vi "Drive Controller.vi"(8 "error in":errorcluster) -> ()   [LabVIEW 2020]
doc: "This VI executes continuously carrying out the current operation and responding to updates or new operation requests. It will often contain the timing or control code that is difficult to place directly in TeleOp. This VI generally opens all sensors and motors and isolates the rest of the robot code from knowing implementation details of how the operations are carried out."
uses:
  <vilib>/Rock Robotics/WPI/Framework/Completion Status.ctl
  Drive Setpoints.ctl
  Drive Operations.ctl
  <vilib>/Rock Robotics/WPI/SafetyOutput/WPI_SafetyOutputConfigMenu.ctl
  <vilib>/Rock Robotics/WPI/RobotDrive/WPI_RobotDriveOpen2MotorWithExistingMotors.vi
  <vilib>/Rock Robotics/Network Tables/NT Write Numeric Array.vi
  <vilib>/Rock Robotics/WPI/ThirdParty/REV Robotics/REVLib/Typedef/Spark MAX Motor Type.ctl
  <vilib>/Rock Robotics/WPI/ThirdParty/REV Robotics/REVLib/Typedef/Spark MAX Idle Mode.ctl
panel:
  in  "Interactive Values":T1
  in  "Buttons":cluster{"Execute Cmd":bool, "Abort Cmd":bool}
  out "Command Timing":cluster{"Start Time (ms)":u32, "Iterations":i32}
  out "Status":T3
  out "Setpoints":T4(graph)
  out "Current\nCmd":string
  # "Tip: The graph shows the motor setpoints. It may also be helpful to observe inputs and sensor values.\nYou may also want to display tuning or debugging controls."
  # "Interactive Command: You may fill in the settings for a command\nand schedule it with the Execute button. You can observe and abort\nany command while fine tuning the code for the controller."
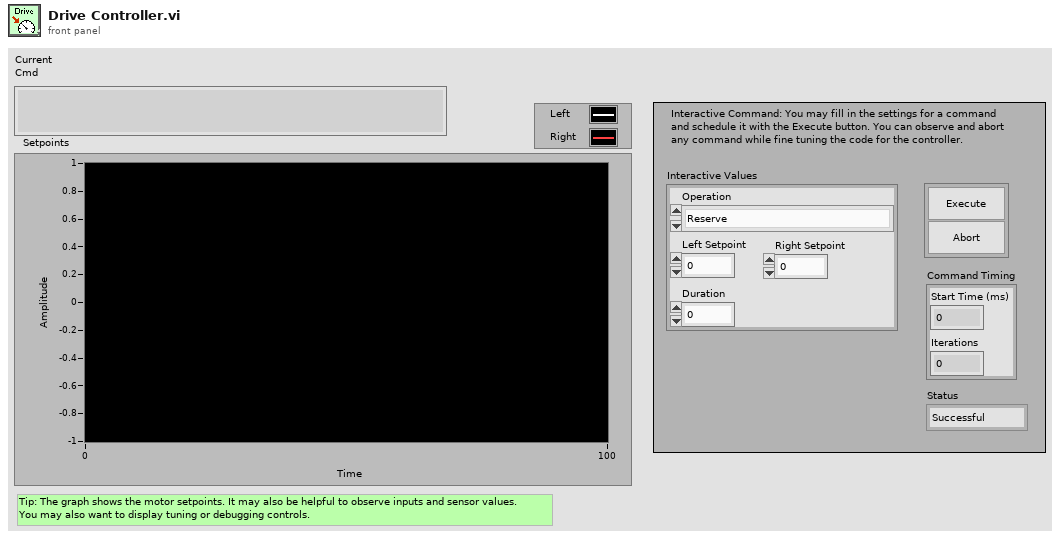
[diagram p1: front panel]
types:
  T1 = typedef "Drive Setpoints.ctl" = cluster{"Operation":T2, "Left Setpoint":dbl, "Right Setpoint":dbl, "Duration":dbl}
  T2 = typedef "Drive Operations.ctl" = enum16{"Reserve", "Read Current", "Immediate", "Drive for Time", "Drive for Distance"}
  T3 = typedef "Completion Status.ctl" = enum16{"Successful", "Aborted", "Incomplete"}
  T4 = cluster{"Left Setpoint":dbl, "Right Setpoint":dbl}
  T5 = typedef "WPI_SafetyOutputConfigMenu.ctl" = enum16{"Enable", "Disable"}
  T6 = typedef "Spark MAX Motor Type.ctl" = enum16{"Brushed", "Brushless"}
  T7 = typedef "Spark MAX Idle Mode.ctl" = enum16{"Coast", "Brake"}
  T8 = typedef "WPI_MotorControlDeviceRef.ctl" = cluster{"DeviceStatus":errorcluster, "Type":T9, "PWM":cluster{"PWM Channel":T10, "DeadBand":T11}, "CAN":cluster{"Device Number":u8, "SetOutput VI Ref":variant, "GetOutput VI Ref":variant, "Enable VI Ref":variant, "Disable VI Ref":variant, "Data":variant}, "Invert":bool, "DIO PWM":cluster{"PWM \"Enable\" Channel":T10, "DIOChannel":T12, "PWM Rate":dbl}}
  T9 = typedef "WPI_MotorControlType.ctl" = enum16{"PWM", "CAN", "DIO PWM"}
  T10 = typedef "FPGA_DIOPWMChannel.ctl" = enum8{"PWM 0", "PWM 1", "PWM 2", "PWM 3", "PWM 4", "PWM 5", "PWM 6", "PWM 7", "PWM 8", "PWM 9", "PWM MXP 0", "PWM MXP 1", "PWM MXP 2", "PWM MXP 3", "PWM MXP 4", "PWM MXP 5", "PWM MXP 6", "PWM MXP 7", "PWM MXP 8", "PWM MXP 9", "Invalid"}
  T11 = typedef "WPI_PWMDeadband.ctl" = cluster{"Name":string, "maxPositivePwm":i32, "minPositivePwm":i32, "centerPwm":i32, "maxNegativePwm":i32, "minNegativePwm":i32, "angularRange":u16}
  T12 = typedef "FPGA_DIOChannel.ctl" = enum8{"DIO 0", "DIO 1", "DIO 2", "DIO 3", "DIO 4", "DIO 5", "DIO 6", "DIO 7", "DIO 8", "DIO 9", "DIO MXP 0", "DIO MXP 1", "DIO MXP 2", "DIO MXP 3", "DIO MXP 4", "DIO MXP 5", "DIO MXP 6", "DIO MXP 7", "DIO MXP 8", "DIO MXP 9", "DIO MXP 10", "DIO MXP 11", "DIO MXP 12", "DIO MXP 13", "DIO MXP 14", "DIO MXP 15", "SPI Port CS1", "SPI Port CS2", "SPI Port CS3", "SPI Port MISO", "SPI Port MOSI", "Invalid"}
  T13 = typedef "WPI_RobotDriveDevRef.ctl" = cluster{"DevStatus":errorcluster, "Motors[]":T8[], "Square Inputs":bool, "Max Output":dbl}
  T14 = typedef "Command Status Info.ctl" = cluster{"Name":string, "Status":T3, "notifier out":T15}
  T15 = typedef "Completion Notifier.ctl" = refnum<notifier>
  T16 = cluster{"SubSystem Data":T1, cluster{"Start Time (ms)":u32, "Iterations":i32}, cluster{"Command Info":T14, "Description":string, "Default Command":T1, "queue out":refnum<queue>, "Subsystem Name":string}}
  T17 = cluster{"SubSystem Data":T1, cluster{"Start Time (ms)":u32, "Iterations":i32}, "Default Command Arguments":cluster{"Command Info":T14, "Description":string, "Default Command":T1, "queue out":refnum<queue>, "Subsystem Name":string}}
  T18 = cluster{"Don't move motors while reserved":dbl, "Don't move motors while reserved":dbl}
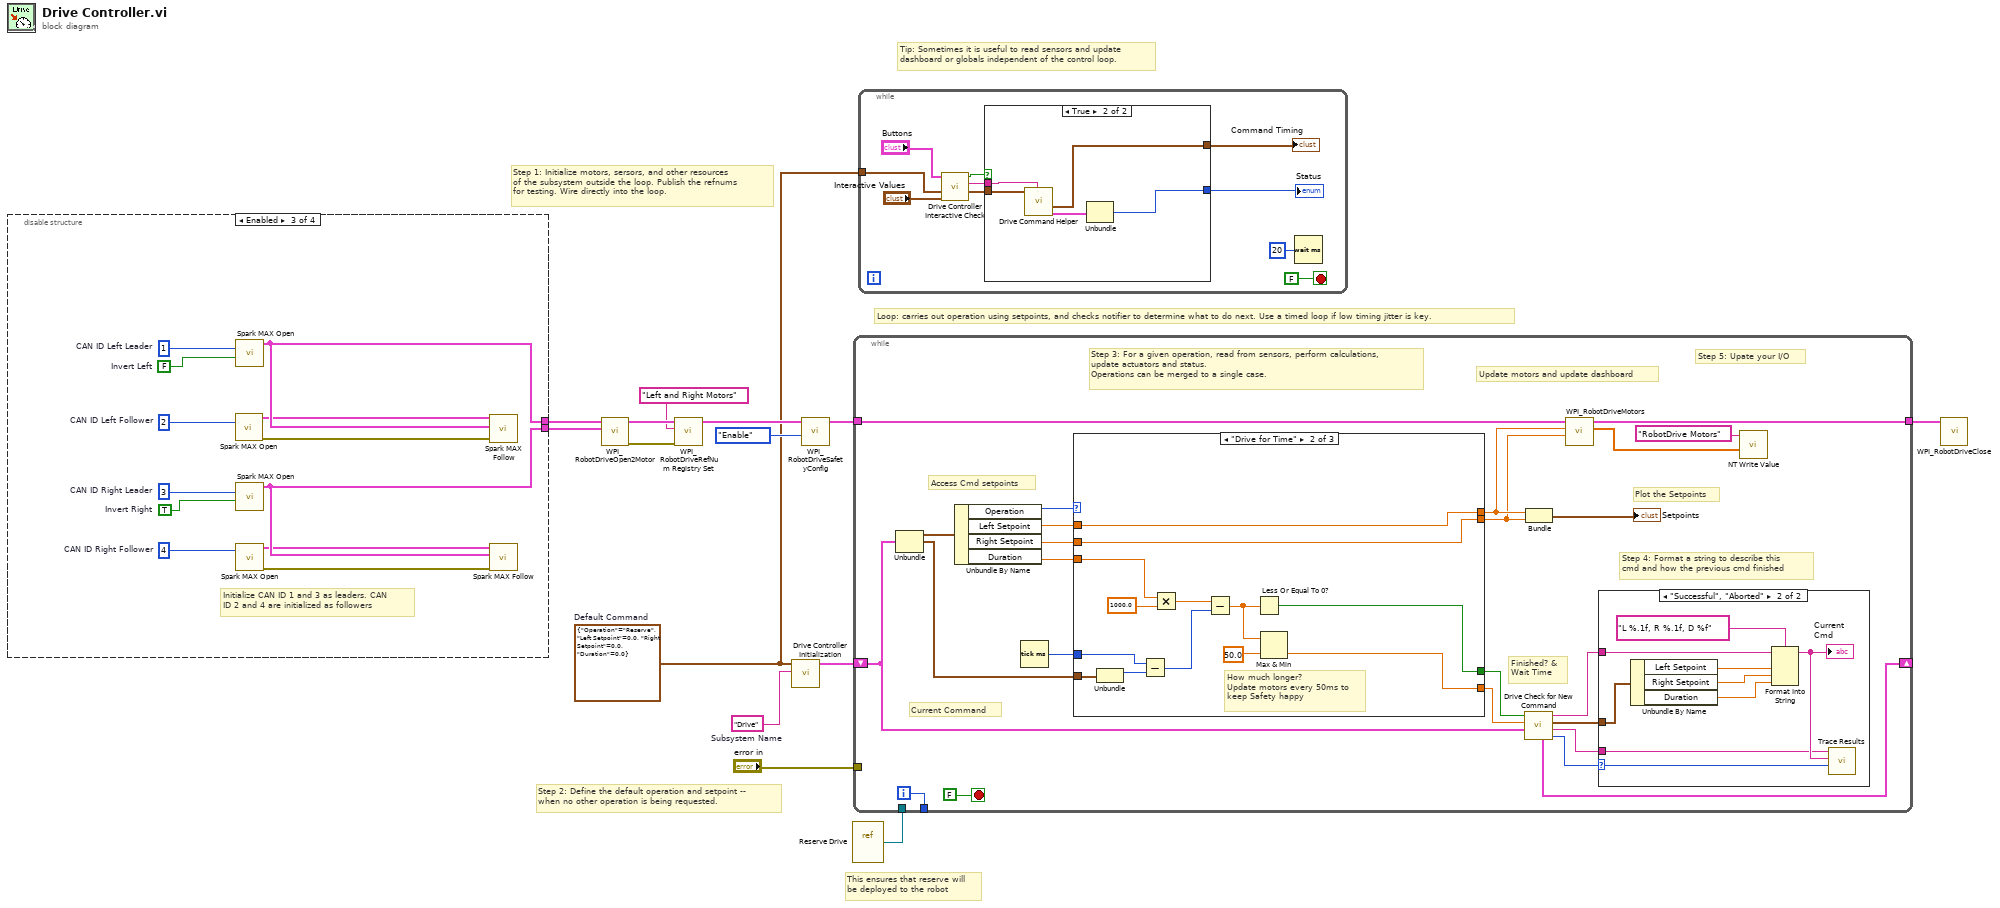
[diagram p0: block diagram]
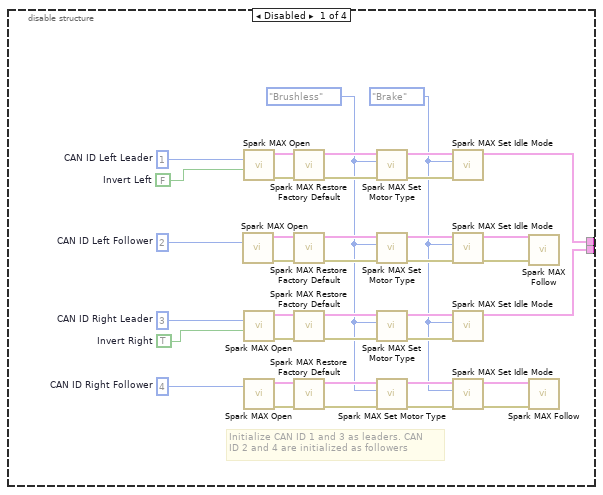
[diagram p2: hidden frame]
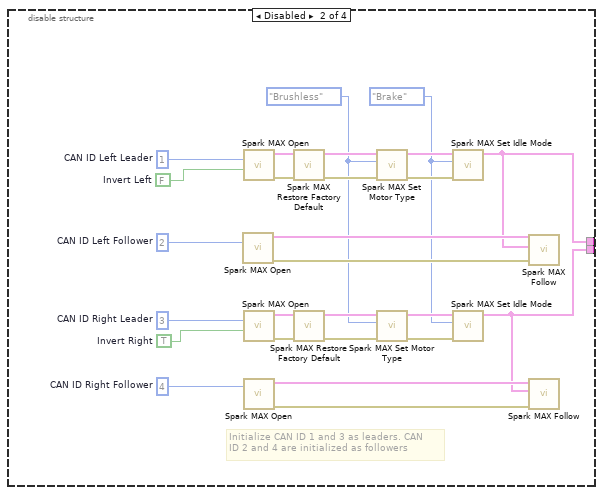
[diagram p3: hidden frame]
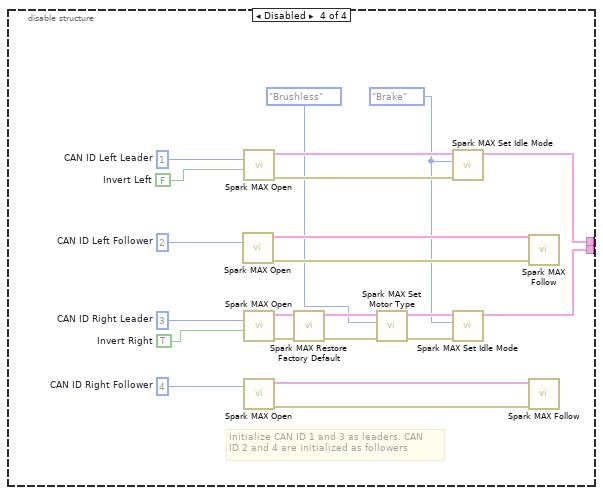
[diagram p4: hidden frame]
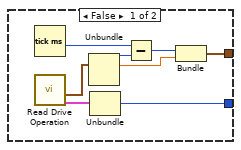
[diagram p5: hidden frame]
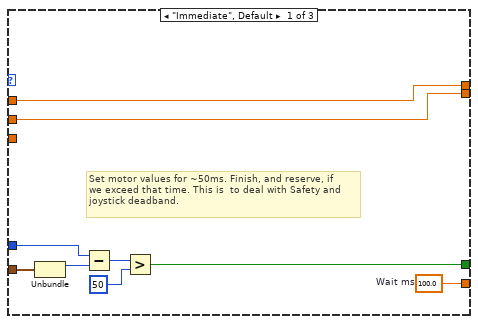
[diagram p7: hidden frame]
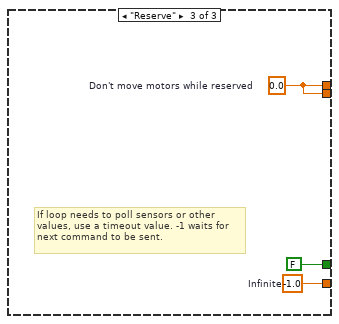
[diagram p8: hidden frame]
diagram:
  w4 = T1 {"Operation"=enum."Reserve", "Left Setpoint"=0.0, "Right Setpoint"=0.0, "Duration"=0.0}  # Default Command
  w14 = "Drive"  # Subsystem Name
  # "This ensures that reserve will\nbe deployed to the robot"
  # "Tip: Sometimes it is useful to read sensors and update\ndashboard or globals independent of the control loop."
  # "Step 2: Define the default operation and setpoint --\nwhen no other operation is being requested."
  # "Step 1: Initialize motors, sersors, and other resources\nof the subsystem outside the loop. Publish the refnums\nfor testing. Wire directly into the loop."
  # "Loop: carries out operation using setpoints, and checks notifier to determine what to do next. Use a timed loop if low timing jitter is key."
  n1 = disable-structure shown="Enabled" {
    disable-tunnel: [w22 w56 w86 w94] -> w3
    disable-tunnel: [w21 w55 w83 w93] -> w2
    frame Disabled {
      w23 = Spark_MAX_Idle_Mode."Brake" ("Idle Mode")
      w32 = Spark_MAX_Motor_Type."Brushless" ("Motor Type")
      w20 = FALSE  # Invert Left
      w19 = TRUE  # Invert Right
      w50 = u8 3  # CAN ID Right Leader
      w49 = u8 4  # CAN ID Right Follower
      w51 = u8 1  # CAN ID Left Leader
      w52 = u8 2  # CAN ID Left Follower
      # "Initialize CAN ID 1 and 3 as leaders. CAN \nID 2 and 4 are initialized as followers"
      n2 = call <vilib>:"Spark MAX Open.vi"("Device Number"=w52) -> ("error out"=w46:errorcluster, "MotorControlDeviceRef"=w45:T8)  [unwired: 9 in]
      n3 = call <vilib>:"Spark MAX Open.vi"("Invert"=w20, "Device Number"=w51) -> ("error out"=w48:errorcluster, "MotorControlDeviceRef"=w47:T8)  [unwired: 8 in]
      n4 = call <vilib>:"Spark MAX Open.vi"("Invert"=w19, "Device Number"=w50) -> ("error out"=w44:errorcluster, "MotorControlDeviceRef"=w43:T8)  [unwired: 8 in]
      n5 = call <vilib>:"Spark MAX Open.vi"("Device Number"=w49) -> ("error out"=w42:errorcluster, "MotorControlDeviceRef"=w41:T8)  [unwired: 9 in]
      n6 = call <vilib>:"Spark MAX Restore Factory Default.vi"("error in"=w48, "MotorControlDeviceRef"=w47) -> ("error out"=w40:errorcluster, "MotorControlDeviceRef"=w39:T8)  [unwired: 8 in]
      n7 = call <vilib>:"Spark MAX Restore Factory Default.vi"("error in"=w46, "MotorControlDeviceRef"=w45) -> ("error out"=w38:errorcluster, "MotorControlDeviceRef"=w37:T8)  [unwired: 8 in]
      n8 = call <vilib>:"Spark MAX Restore Factory Default.vi"("error in"=w44, "MotorControlDeviceRef"=w43) -> ("error out"=w36:errorcluster, "MotorControlDeviceRef"=w35:T8)  [unwired: 8 in]
      n9 = call <vilib>:"Spark MAX Restore Factory Default.vi"("error in"=w42, "MotorControlDeviceRef"=w41) -> ("error out"=w34:errorcluster, "MotorControlDeviceRef"=w33:T8)  [unwired: 8 in]
      n10 = call <vilib>:"Spark MAX Set Motor Type.vi"("error in (no error)"=w40, "Motor Type"=w32, "MotorControlDevRef"=w39) -> ("error out"=w31:errorcluster, "MotorControlDeviceRef"=w30:T8)  [unwired: 7 in]
      n11 = call <vilib>:"Spark MAX Set Motor Type.vi"("error in (no error)"=w38, "Motor Type"=w32, "MotorControlDevRef"=w37) -> ("error out"=w29:errorcluster, "MotorControlDeviceRef"=w28:T8)  [unwired: 7 in]
      n12 = call <vilib>:"Spark MAX Set Motor Type.vi"("error in (no error)"=w36, "Motor Type"=w32, "MotorControlDevRef"=w35) -> ("error out"=w27:errorcluster, "MotorControlDeviceRef"=w26:T8)  [unwired: 7 in]
      n13 = call <vilib>:"Spark MAX Set Motor Type.vi"("error in (no error)"=w34, "Motor Type"=w32, "MotorControlDevRef"=w33) -> ("error out"=w25:errorcluster, "MotorControlDeviceRef"=w24:T8)  [unwired: 7 in]
      n14 = call <vilib>:"Spark MAX Set Idle Mode.vi"("error in (no error)"=w31, "Idle Mode"=w23, "MotorControlDeviceRef in"=w30) -> ("MotorControlDeviceRef out"=w22:T8)  [unwired: 7 in, 1 out]
      n15 = call <vilib>:"Spark MAX Set Idle Mode.vi"("error in (no error)"=w29, "Idle Mode"=w23, "MotorControlDeviceRef in"=w28) -> ("error out"=w18:errorcluster, "MotorControlDeviceRef out"=w17:T8)  [unwired: 7 in]
      n16 = call <vilib>:"Spark MAX Set Idle Mode.vi"("error in (no error)"=w27, "Idle Mode"=w23, "MotorControlDeviceRef in"=w26) -> ("MotorControlDeviceRef out"=w21:T8)  [unwired: 7 in, 1 out]
      n17 = call <vilib>:"Spark MAX Set Idle Mode.vi"("error in (no error)"=w25, "Idle Mode"=w23, "MotorControlDeviceRef in"=w24) -> ("error out"=w16:errorcluster, "MotorControlDeviceRef out"=w15:T8)  [unwired: 7 in]
      n18 = call <vilib>:"Spark MAX Follow.vi"("error in (no error)"=w18, "MotorControlDeviceRef"=w17) -> ()  [unwired: 8 in, 2 out]
      n19 = call <vilib>:"Spark MAX Follow.vi"("error in (no error)"=w16, "MotorControlDeviceRef"=w15) -> ()  [unwired: 8 in, 2 out]
    }
    frame Disabled {
      w57 = Spark_MAX_Idle_Mode."Brake" ("Idle Mode")
      w62 = Spark_MAX_Motor_Type."Brushless" ("Motor Type")
      w54 = FALSE  # Invert Left
      w53 = TRUE  # Invert Right
      w76 = u8 3  # CAN ID Right Leader
      w75 = u8 4  # CAN ID Right Follower
      w77 = u8 1  # CAN ID Left Leader
      w78 = u8 2  # CAN ID Left Follower
      # "Initialize CAN ID 1 and 3 as leaders. CAN \nID 2 and 4 are initialized as followers"
      n20 = call <vilib>:"Spark MAX Open.vi"("Device Number"=w78) -> ("error out"=w68:errorcluster, "MotorControlDeviceRef"=w67:T8)  [unwired: 9 in]
      n21 = call <vilib>:"Spark MAX Open.vi"("Invert"=w54, "Device Number"=w77) -> ("error out"=w74:errorcluster, "MotorControlDeviceRef"=w73:T8)  [unwired: 8 in]
      n22 = call <vilib>:"Spark MAX Open.vi"("Invert"=w53, "Device Number"=w76) -> ("error out"=w72:errorcluster, "MotorControlDeviceRef"=w71:T8)  [unwired: 8 in]
      n23 = call <vilib>:"Spark MAX Open.vi"("Device Number"=w75) -> ("error out"=w64:errorcluster, "MotorControlDeviceRef"=w63:T8)  [unwired: 9 in]
      n24 = call <vilib>:"Spark MAX Restore Factory Default.vi"("error in"=w74, "MotorControlDeviceRef"=w73) -> ("error out"=w70:errorcluster, "MotorControlDeviceRef"=w69:T8)  [unwired: 8 in]
      n25 = call <vilib>:"Spark MAX Restore Factory Default.vi"("error in"=w72, "MotorControlDeviceRef"=w71) -> ("error out"=w66:errorcluster, "MotorControlDeviceRef"=w65:T8)  [unwired: 8 in]
      n26 = call <vilib>:"Spark MAX Set Motor Type.vi"("error in (no error)"=w70, "Motor Type"=w62, "MotorControlDevRef"=w69) -> ("error out"=w61:errorcluster, "MotorControlDeviceRef"=w60:T8)  [unwired: 7 in]
      n27 = call <vilib>:"Spark MAX Set Motor Type.vi"("error in (no error)"=w66, "Motor Type"=w62, "MotorControlDevRef"=w65) -> ("error out"=w59:errorcluster, "MotorControlDeviceRef"=w58:T8)  [unwired: 7 in]
      n28 = call <vilib>:"Spark MAX Set Idle Mode.vi"("error in (no error)"=w61, "Idle Mode"=w57, "MotorControlDeviceRef in"=w60) -> ("MotorControlDeviceRef out"=w56:T8)  [unwired: 7 in, 1 out]
      n29 = call <vilib>:"Spark MAX Set Idle Mode.vi"("error in (no error)"=w59, "Idle Mode"=w57, "MotorControlDeviceRef in"=w58) -> ("MotorControlDeviceRef out"=w55:T8)  [unwired: 7 in, 1 out]
      n30 = call <vilib>:"Spark MAX Follow.vi"("error in (no error)"=w68, "Master Controller"=w56, "MotorControlDeviceRef"=w67) -> ()  [unwired: 7 in, 2 out]
      n31 = call <vilib>:"Spark MAX Follow.vi"("error in (no error)"=w64, "Master Controller"=w55, "MotorControlDeviceRef"=w63) -> ()  [unwired: 7 in, 2 out]
    }
    frame Enabled {
      w80 = FALSE  # Invert Left
      w79 = TRUE  # Invert Right
      w88 = u8 3  # CAN ID Right Leader
      w87 = u8 4  # CAN ID Right Follower
      w89 = u8 1  # CAN ID Left Leader
      w90 = u8 2  # CAN ID Left Follower
      # "Initialize CAN ID 1 and 3 as leaders. CAN \nID 2 and 4 are initialized as followers"
      n32 = call <vilib>:"Spark MAX Open.vi"("Device Number"=w90) -> ("error out"=w85:errorcluster, "MotorControlDeviceRef"=w84:T8)  [unwired: 9 in]
      n33 = call <vilib>:"Spark MAX Open.vi"("Invert"=w80, "Device Number"=w89) -> ("MotorControlDeviceRef"=w86:T8)  [unwired: 8 in, 1 out]
      n34 = call <vilib>:"Spark MAX Open.vi"("Invert"=w79, "Device Number"=w88) -> ("MotorControlDeviceRef"=w83:T8)  [unwired: 8 in, 1 out]
      n35 = call <vilib>:"Spark MAX Open.vi"("Device Number"=w87) -> ("error out"=w82:errorcluster, "MotorControlDeviceRef"=w81:T8)  [unwired: 9 in]
      n36 = call <vilib>:"Spark MAX Follow.vi"("error in (no error)"=w85, "Master Controller"=w86, "MotorControlDeviceRef"=w84) -> ()  [unwired: 7 in, 2 out]
      n37 = call <vilib>:"Spark MAX Follow.vi"("error in (no error)"=w82, "Master Controller"=w83, "MotorControlDeviceRef"=w81) -> ()  [unwired: 7 in, 2 out]
    }
    frame Disabled {
      w95 = Spark_MAX_Idle_Mode."Brake" ("Idle Mode")
      w92 = FALSE  # Invert Left
      w91 = TRUE  # Invert Right
      w110 = u8 3  # CAN ID Right Leader
      w109 = u8 4  # CAN ID Right Follower
      w111 = u8 1  # CAN ID Left Leader
      w112 = u8 2  # CAN ID Left Follower
      # "Initialize CAN ID 1 and 3 as leaders. CAN \nID 2 and 4 are initialized as followers"
      n38 = call <vilib>:"Spark MAX Open.vi"("Device Number"=w112) -> ("error out"=w104:errorcluster, "MotorControlDeviceRef"=w103:T8)  [unwired: 9 in]
      n39 = call <vilib>:"Spark MAX Open.vi"("Invert"=w92, "Device Number"=w111) -> ("error out"=w106:errorcluster, "MotorControlDeviceRef"=w105:T8)  [unwired: 8 in]
      n40 = call <vilib>:"Spark MAX Open.vi"("Invert"=w91, "Device Number"=w110) -> ("error out"=w108:errorcluster, "MotorControlDeviceRef"=w107:T8)  [unwired: 8 in]
      n41 = call <vilib>:"Spark MAX Open.vi"("Device Number"=w109) -> ("error out"=w100:errorcluster, "MotorControlDeviceRef"=w99:T8)  [unwired: 9 in]
      n42 = call <vilib>:"Spark MAX Restore Factory Default.vi"("error in"=w108, "MotorControlDeviceRef"=w107) -> ("error out"=w102:errorcluster, "MotorControlDeviceRef"=w101:T8)  [unwired: 8 in]
      n43 = call <vilib>:"Spark MAX Set Motor Type.vi"("error in (no error)"=w102, "Motor Type"=Spark_MAX_Motor_Type."Brushless", "MotorControlDevRef"=w101) -> ("error out"=w97:errorcluster, "MotorControlDeviceRef"=w96:T8)  [unwired: 7 in]
      n44 = call <vilib>:"Spark MAX Set Idle Mode.vi"("error in (no error)"=w106, "Idle Mode"=w95, "MotorControlDeviceRef in"=w105) -> ("MotorControlDeviceRef out"=w94:T8)  [unwired: 7 in, 1 out]
      n45 = call <vilib>:"Spark MAX Set Idle Mode.vi"("error in (no error)"=w97, "Idle Mode"=w95, "MotorControlDeviceRef in"=w96) -> ("MotorControlDeviceRef out"=w93:T8)  [unwired: 7 in, 1 out]
      n46 = call <vilib>:"Spark MAX Follow.vi"("error in (no error)"=w104, "MotorControlDeviceRef"=w103) -> ()  [unwired: 8 in, 2 out]
      n47 = call <vilib>:"Spark MAX Follow.vi"("error in (no error)"=w100, "MotorControlDeviceRef"=w99) -> ()  [unwired: 8 in, 2 out]
    }
  }
  n48 = call-poly <vilib>:"WPI_RobotDriveOpen2Motor.vi"("Right Motor Dev Ref"=w2, "Left Motor Dev Ref"=w3) -> ("error out"=w11:errorcluster, "RobotDriveDevRef"=w13:T13)  [unwired: 3 in, 5 out]
  n49 = call <vilib>:"WPI_RobotDriveRefNum Registry Set.vi"("error in (no error)"=w11, "refnum name"="Left and Right Motors", "RobotDriveDevRef"=w13) -> ("RobotDriveDevRef"=w10:T13)  [unwired: 1 in, 7 out]
  n50 = call "Drive Controller Initialization.vi"("Subsystem Name"=w14, "Default Command"=w4) -> ("Current Command"=w6:T16)  [unwired: 9 in]
  n51 = call <vilib>:"WPI_RobotDriveSafetyConfig.vi"("mode"=WPI_SafetyOutputConfigMenu."Enable", "RobotDriveDevRef"=w10) -> ("RobotDriveDevRef"=w8:T13)  [unwired: 8 in, 1 out]
  n52 = vi-ref "Reserve Drive.vi"() -> (w5:refnum<vi>)
  n53 = while {
    shift-right: [w123] -> _
    shift-left: w6 -> [w116]
    tunnel: [w135] -> _
    tunnel: w8 -> [w131]
    tunnel: "error in" -> [_]
    tunnel: w5 -> [_]
    tunnel: [w115] -> w1
    i -> [w135]
    stop <- FALSE stop-if-true
    # "Step 5: Upate your I/O"
    # "Step 4: Format a string to describe this\ncmd and how the previous cmd finished"
    # "Current Command"
    # "Update motors and update dashboard"
    # "Plot the Setpoints"
    # "Access Cmd setpoints"
    # "Finished? &\nWait Time"
    # "Step 3: For a given operation, read from sensors, perform calculations,\nupdate actuators and status.\nOperations can be merged to a single case."
    n54 = Unbundle(w116) -> ("SubSystem Data"=w130:T1, w117:cluster{"Start Time (ms)":u32, "Iterations":i32})  [unwired: 1 out]
    n55 = Unbundle By Name(w130) -> ("Operation"=w129:T2, "Left Setpoint"=w128:dbl, "Right Setpoint"=w127:dbl, "Duration"=w126:dbl)
    n56 = Tick Count (ms)() -> (millisecond timer value=w125:u32)
    n57 = case shown="\"Drive for Time\"" w129 {
      tunnel: [w154 w155 w170] -> w122
      tunnel: [w147 w162 FALSE ("ignore previous (F)")] -> w121
      tunnel: w117 -> [w146 w164 _]
      tunnel: [w153 w161 w168] -> w133
      tunnel: [w152 w160 w168] -> w132
      tunnel: w128 -> [w153 w161 _]
      tunnel: w127 -> [w152 w160 _]
      tunnel: w126 -> [_ w159 _]
      tunnel: w125 -> [w148 w158 _]
      frame "Immediate", Default {
        w154 = 100.0  # Wait ms
        # "Set motor values for ~50ms. Finish, and reserve, if\nwe exceed that time. This is  to deal with Safety and\njoystick deadband."
        n58 = Unbundle(w146) -> ("Start Time (ms)"=w149:u32)  [unwired: 1 out]
        n59 = Subtract(x=w148, y=w149) -> (x-y=w150:u32)
        n60 = Greater?(x=w150, y=u8 50 ("Left Motor")) -> (0:w147:bool)
      }
      frame "Drive for Time" {
        # "How much longer?\nUpdate motors every 50ms to\nkeep Safety happy"
        n61 = Unbundle(w164) -> ("Start Time (ms)"=w163:u32)  [unwired: 1 out]
        n62 = Subtract(x=w158, y=w163) -> (x-y=w167:u32)
        n63 = Multiply(x=w159, y=1000.0) -> (x*y=w166:dbl)
        n64 = Subtract(x=w166, y=w167) -> (x-y=w157:dbl)
        n65 = Less Or Equal To 0?(x=w157) -> (x <= 0?=w162:bool)
        n66 = Max & Min(x=w157, y=50.0) -> (min(x,y)=w155:dbl)  [unwired: 1 out]
      }
      frame "Reserve" {
        w168 = 0.0  # Don't move motors while reserved
        w170 = -1.0  # Infinite
        # "If loop needs to poll sensors or other\nvalues, use a timeout value. -1 waits for\nnext command to be sent."
      }
    }
    n67 = call "Drive Check for New Command.vi"("input cluster"=w116, "Wait time (ms)"=w122, "Finished?"=w121) -> ("Completion"=w124:T3, "Subsystem Name"=w118:string, "Current Command"=w119:T1, "Initial Trace String"=w120:string, "Next Command"=w123:T17)  [unwired: 4 in]
    n68 = Bundle("Don't move motors while reserved"=w133, "Don't move motors while reserved"=w132) -> (→"Setpoints":T18)  [unwired: 1 in]
    n69 = call <vilib>:"WPI_RobotDriveMotors.vi"("RightSpeed"=w132, "LeftSpeed"=w133, "RobotDriveDevRef"=w131) -> ("Motor Values"=w114:dbl[], "RobotDriveDevRef"=w115:T13)  [unwired: 1 in, 6 out]
    n70 = case shown="\"Successful\", \"Aborted\"" w124 {
      selector: w124 -> [_ w145]
      tunnel: w120 -> [_ w140]
      tunnel: w119 -> [_ w141]
      tunnel: w118 -> [_ w137]
      frame "Incomplete", Default {
        # "Continuing current command"
      }
      frame "Successful", "Aborted" {
        # "Report and setup for next command"
        n71 = Unbundle By Name(w141) -> ("Left Setpoint"=w143:dbl, "Right Setpoint"=w144:dbl, "Duration"=w138:dbl)
        n72 = Format Into String(format string="L %.1f, R %.1f, D %f", initial string=w140, w143, w144, w138) -> (resulting string=w139:string)  [unwired: 1 in, 1 out]
        "Current\nCmd" <- w139
        n73 = call <vilib>:"Trace Results.vi"("Status of previous command"=w145, "Description"=w139, "Subsystem"=w137) -> ()  [unwired: 9 in]
      }
    }
    n74 = call-poly <vilib>:"NT Write Value.vi"("Numeric Array"=w114, "Name"="RobotDrive Motors") -> ()  [unwired: 9 in, 1 out]
  }
  n75 = while {
    tunnel: w4 -> [w172]
    stop <- FALSE stop-if-true
    n76 = call "Drive Controller Interactive Check.vi"("Interactive Command In"="Interactive Values", "Default Command"=w172, "Buttons"="Buttons") -> ("Interactive Command Out"=w174:T1, "Trace String"=w175:string, "Schedule"=w176:bool)  [unwired: 6 in]
    n77 = case shown="True" w176 {
      tunnel: [w185 w193] -> w177
      tunnel: [w184 w189] -> w178
      tunnel: w175 -> [_ w191]
      tunnel: w174 -> [_ w190]
      frame False {
        n78 = Tick Count (ms)() -> (millisecond timer value=w188:u32)
        n79 = call "Read Drive Operation.vi"() -> ("Command Info"=w182:T14, "SubSystem Data"=w181:T1)  [unwired: 9 in, 1 out]
        n80 = Unbundle(w181) -> ("Operation"=w186:T2, "Left Setpoint"=w183:dbl)  [unwired: 2 out]
        n81 = Unbundle(w182) -> ("Status"=w185:T3)  [unwired: 2 out]
        n82 = Subtract(x=w188, y=w186) -> (x-y=w187:u32)
        n83 = Bundle(w187, "Left Setpoint"=w183) -> (w184:cluster{u32, "Left Setpoint":dbl})  [unwired: 1 in]
      }
      frame True {
        n84 = call "Drive Command Helper.vi"("Description"=w191, "SubSystem Data"=w190) -> ("Command Info Out"=w192:T14, "Command Timing"=w189:cluster{"Start Time (ms)":u32, "Iterations":i32})  [unwired: 7 in, 1 out]
        n85 = Unbundle(w192) -> ("Status"=w193:T3)  [unwired: 2 out]
      }
    }
    "Status" <- w177
    "Command Timing" <- w178
    n86 = Wait (ms)(milliseconds to wait=u32 20) -> ()  [unwired: 1 out]
  }
  n87 = call <vilib>:"WPI_RobotDriveClose.vi"("RobotDriveDevRef"=w1) -> ()  [unwired: 10 in, 1 out]
